vi "AC mVolt Configuration.vi"(8 "error in (no error)":errorcluster, 10 "mVoltage Range":T1, 11 "VISA resource name":refnum<visa-resource-name>) -> (0 "error out":errorcluster, 3 "VISA resource name out":refnum<visa-resource-name>)   [LabVIEW 2015, in "Keysight U1252.lvlib"]
uses:
  <instrlib>/Keysight U1252/Keysight U1252.lvlib
  <instrlib>/Keysight U1252/Controls/Mili Votalge Range.ctl
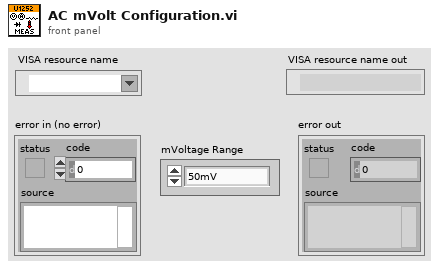
[diagram p1: front panel]
types:
  T1 = typedef "Keysight U1252.lvlib/Mili Votalge Range.ctl" = enum16{"50mV", "500mV", "1000mV", "Auto"}
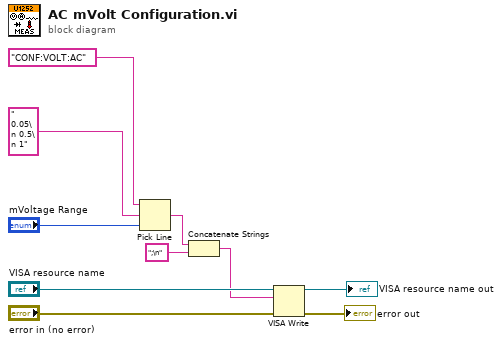
[diagram p0: block diagram]
diagram:
  n1 = Pick Line(string ("")="CONF:VOLT:AC", multi-line string=" 0.05\n 0.5\n 1", line index="mVoltage Range") -> (output string=w4:string)
  n2 = Concatenate Strings(w4, ";\n" ("string")) -> (w2:string)
  n3 = VISA Write(VISA resource name="VISA resource name", write buffer=w2, error in (no error)="error in (no error)") -> (VISA resource name out=→"VISA resource name out":refnum<visa-resource-name>, error out=→"error out":errorcluster)  [unwired: 1 out]
